vi "ANA IN Lesen.vi"() -> (0 "Rohwerte":sgl[](array[numeric]), 1 "Istwerte":sgl[](array[numeric]), 3 "Fühlerbruch":bool[](array[boolean]))   [LabVIEW 2020, in "Verwaltung - cRIO.lvlib"]
uses:
  Verwaltung - cRIO.lvlib
  Konfig-Dateien/FGV Betriebsdaten Aktionen.ctl
  Allgemein/FGV FT-IR Kuehlung Aktionen.ctl
  Allgemein/Allgemein.lvlib
  Konfig-Dateien/Konfig-Dateien.lvlib
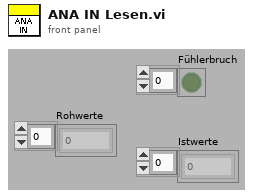
[diagram p1: front panel]
types:
  T1 = typedef "Allgemein.lvlib/FGV FT-IR Kuehlung Aktionen.ctl" = enum16{"lesen", "Kühlung?"}
  T2 = typedef "Konfig-Dateien.lvlib/FGV Betriebsdaten Aktionen.ctl" = enum16{"lesen", "Anlagengrenzw.", "PID Param.", "Sonstige", "Sensor Para."}
  T3 = typedef "Erweiterte Konfig.lvlib/Parameter Sensoren.ctl" = cluster{"Kal.Durchfl.FTIR":sgl, "Kal.Durchfl.PMA":sgl, "Offset Durchfl.FTIR":sgl, "Offset Druck Ausgang":sgl, "Offset Druck Umgebung":sgl, "Offset Durchfl.PMA":sgl, "Offset Druck CG PMA":sgl, "Offset Druck CG":sgl, "Offset Druck FTIR IAG":sgl, "Druck Kalter Block":sgl}
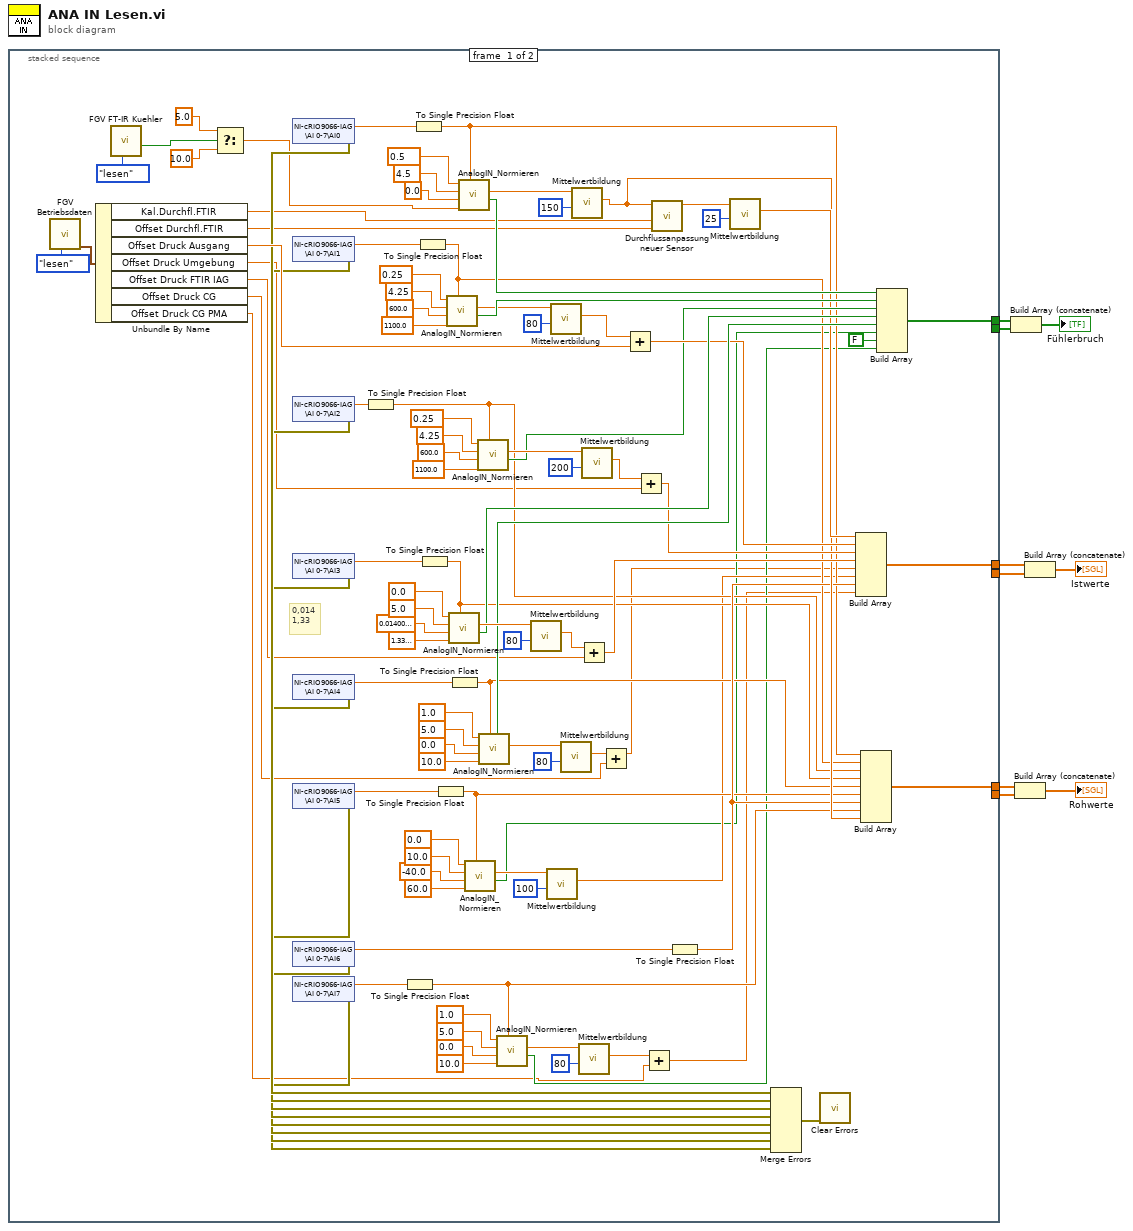
[diagram p0: block diagram]
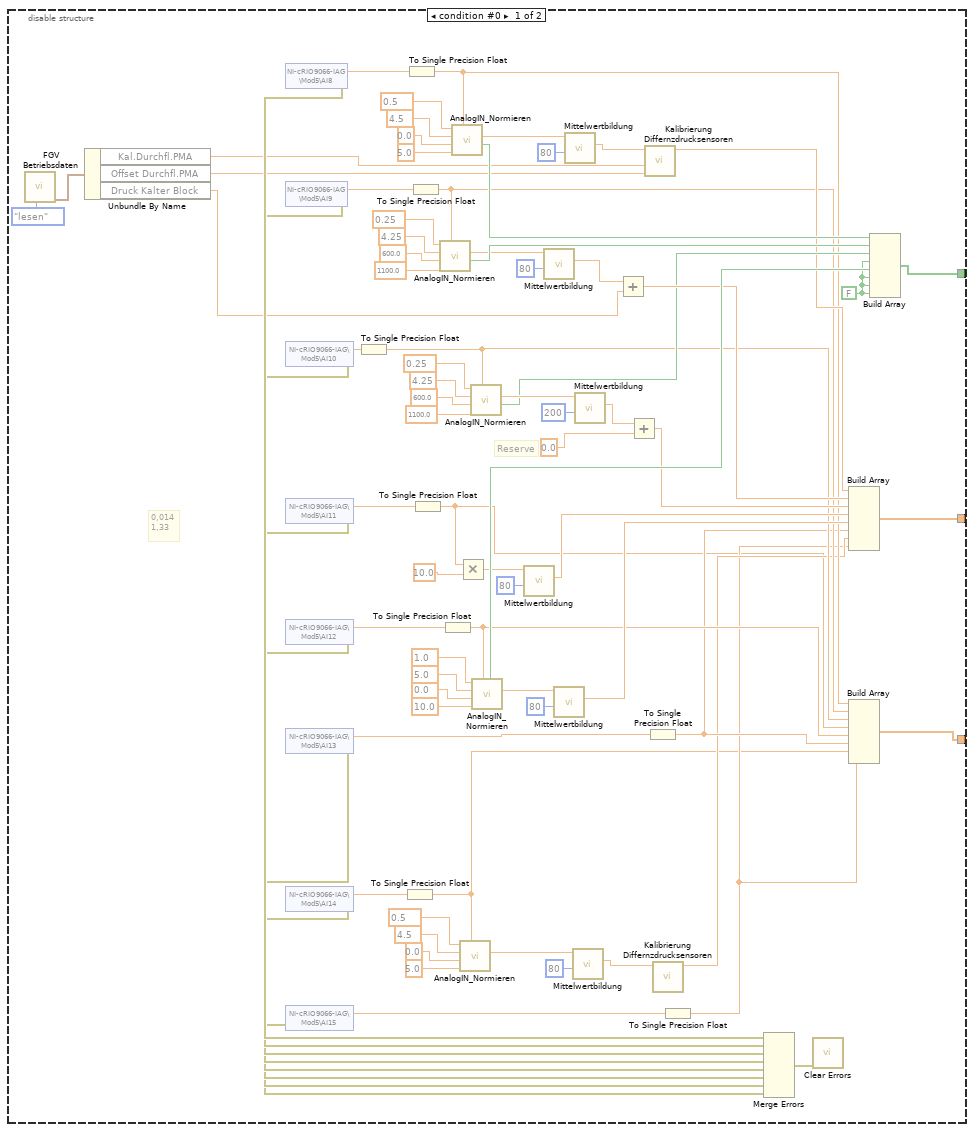
[diagram p3: hidden frame]
diagram:
  n1 = stacked-sequence {
    tunnel: [w50 _] -> w9
    tunnel: [_ w118] -> w8
    tunnel: [w49 _] -> w7
    tunnel: [_ w117] -> w6
    tunnel: [w42 _] -> w2
    tunnel: [_ w116] -> w3
    frame #0 {
      # "0,014\n1,33"
      n2 = call "FGV Betriebsdaten.vi"("Aktionen"=FGV_Betriebsdaten_Aktionen."lesen") -> ("Parameter Sensoren"=w21:T3)  [unwired: 7 in, 3 out]
      n3 = Unbundle By Name(w21) -> ("Kal.Durchfl.FTIR"=w55:sgl, "Offset Durchfl.FTIR"=w54:sgl, "Offset Druck Ausgang"=w77:sgl, "Offset Druck Umgebung"=w20:sgl, "Offset Druck FTIR IAG"=w19:sgl, "Offset Druck CG"=w17:sgl, "Offset Druck CG PMA"=w15:sgl)
      n4 = call "FGV FT-IR Kuehler.vi"("Aktionen"=FGV_FT-IR_Kuehlung_Aktionen."lesen") -> ("Durchflusssensor 0-5V"=w11:bool)  [unwired: 6 in, 4 out]
      n5 = Select(t=sgl 5.0 ("Obergrenze"), s=w11, f=sgl 10.0 ("Obergrenze")) -> (s? t:f=w10:sgl)
      n6 = shared-variable "NI-cRIO9066-IAG\\AI 0-7\\AI0"() -> (w101:dbl, error out=w73:errorcluster)  [unwired: 1 in]
      n7 = shared-variable "NI-cRIO9066-IAG\\AI 0-7\\AI1"() -> (w100:dbl, error out=w72:errorcluster)  [unwired: 1 in]
      n8 = shared-variable "NI-cRIO9066-IAG\\AI 0-7\\AI2"() -> (w99:dbl, error out=w71:errorcluster)  [unwired: 1 in]
      n9 = shared-variable "NI-cRIO9066-IAG\\AI 0-7\\AI3"() -> (w97:dbl, error out=w70:errorcluster)  [unwired: 1 in]
      n10 = shared-variable "NI-cRIO9066-IAG\\AI 0-7\\AI4"() -> (w85:dbl, error out=w69:errorcluster)  [unwired: 1 in]
      n11 = shared-variable "NI-cRIO9066-IAG\\AI 0-7\\AI5"() -> (w35:dbl, error out=w68:errorcluster)  [unwired: 1 in]
      n12 = shared-variable "NI-cRIO9066-IAG\\AI 0-7\\AI6"() -> (w83:dbl, error out=w67:errorcluster)  [unwired: 1 in]
      n13 = shared-variable "NI-cRIO9066-IAG\\AI 0-7\\AI7"() -> (w82:dbl, error out=w66:errorcluster)  [unwired: 1 in]
      n14 = To Single Precision Float(number=w99) -> (single precision float=w45:sgl)
      n15 = To Single Precision Float(number=w82) -> (single precision float=w25:sgl)
      n16 = To Single Precision Float(number=w101) -> (single precision float=w43:sgl)
      n17 = To Single Precision Float(number=w100) -> (single precision float=w44:sgl)
      n18 = To Single Precision Float(number=w97) -> (single precision float=w46:sgl)
      n19 = To Single Precision Float(number=w35) -> (single precision float=w34:sgl)
      n20 = call "AnalogIN_Normieren.vi"("Analogwert"=w44, "Obergrenze"=sgl 1100.0, "Untergrenze"=sgl 600.0, "Max Analogwert"=sgl 4.25, "Min Analogwert"=sgl 0.25) -> ("Unterlauf oder Drahtbruch"=w115:bool, "Normierter Wert"=w102:sgl)  [unwired: 5 out]
      n21 = call "AnalogIN_Normieren.vi"("Analogwert"=w46, "Obergrenze"=sgl 1.33 ("Max Analogwert"), "Untergrenze"=sgl 0.014 ("Min Analogwert"), "Max Analogwert"=sgl 5.0, "Min Analogwert"=sgl 0.0) -> ("Unterlauf oder Drahtbruch"=w81:bool, "Normierter Wert"=w92:sgl)  [unwired: 5 out]
      n22 = To Single Precision Float(number=w85) -> (single precision float=w33:sgl)
      n23 = call "AnalogIN_Normieren.vi"("Analogwert"=w43, "Obergrenze"=w10, "Untergrenze"=sgl 0.0, "Max Analogwert"=sgl 4.5, "Min Analogwert"=sgl 0.5) -> ("Unterlauf oder Drahtbruch"=w114:bool, "Normierter Wert"=w103:sgl)  [unwired: 5 out]
      n24 = call "AnalogIN_Normieren.vi"("Analogwert"=w34, "Obergrenze"=sgl 60.0 ("Max Analogwert"), "Untergrenze"=sgl -40.0 ("Min Analogwert"), "Max Analogwert"=sgl 10.0, "Min Analogwert"=sgl 0.0) -> ("Unterlauf oder Drahtbruch"=w23:bool, "Normierter Wert"=w36:sgl)  [unwired: 5 out]
      n25 = call "AnalogIN_Normieren.vi"("Analogwert"=w45, "Obergrenze"=sgl 1100.0, "Untergrenze"=sgl 600.0, "Max Analogwert"=sgl 4.25, "Min Analogwert"=sgl 0.25) -> ("Unterlauf oder Drahtbruch"=w58:bool, "Normierter Wert"=w64:sgl)  [unwired: 5 out]
      n26 = call "AnalogIN_Normieren.vi"("Analogwert"=w33, "Obergrenze"=sgl 10.0 ("Max Analogwert"), "Untergrenze"=sgl 0.0 ("Min Analogwert"), "Max Analogwert"=sgl 5.0, "Min Analogwert"=sgl 1.0) -> ("Unterlauf oder Drahtbruch"=w80:bool, "Normierter Wert"=w91:sgl)  [unwired: 5 out]
      n27 = call "AnalogIN_Normieren.vi"("Analogwert"=w25, "Obergrenze"=sgl 10.0 ("Max Analogwert"), "Untergrenze"=sgl 0.0 ("Min Analogwert"), "Max Analogwert"=sgl 5.0, "Min Analogwert"=sgl 1.0) -> ("Unterlauf oder Drahtbruch"=w22:bool, "Normierter Wert"=w27:sgl)  [unwired: 5 out]
      n28 = call "Mittelwertbildung.vi"("Anzahl Werte"=u8 80, "Neuer Wert"=w92) -> ("gemittelter Wert"=w76:sgl)  [unwired: 7 in, 2 out]
      n29 = call "Mittelwertbildung.vi"("Anzahl Werte"=u8 100, "Neuer Wert"=w36) -> ("gemittelter Wert"=w24:sgl)  [unwired: 7 in, 2 out]
      n30 = call "Mittelwertbildung.vi"("Anzahl Werte"=u8 80, "Neuer Wert"=w102) -> ("gemittelter Wert"=w79:sgl)  [unwired: 7 in, 2 out]
      n31 = call "Mittelwertbildung.vi"("Anzahl Werte"=u8 80, "Neuer Wert"=w91) -> ("gemittelter Wert"=w84:sgl)  [unwired: 7 in, 2 out]
      n32 = call "Mittelwertbildung.vi"("Anzahl Werte"=u8 150, "Neuer Wert"=w103) -> ("gemittelter Wert"=w48:sgl)  [unwired: 7 in, 2 out]
      n33 = Add(x=w76, y=w19) -> (x+y=w75:sgl)
      n34 = call "Mittelwertbildung.vi"("Anzahl Werte"=u8 80, "Neuer Wert"=w27) -> ("gemittelter Wert"=w26:sgl)  [unwired: 7 in, 2 out]
      n35 = call "Mittelwertbildung.vi"("Anzahl Werte"=u8 200, "Neuer Wert"=w64) -> ("gemittelter Wert"=w57:sgl)  [unwired: 7 in, 2 out]
      n36 = Add(x=w84, y=w17) -> (x+y=w18:sgl)
      n37 = Add(x=w79, y=w77) -> (x+y=w78:sgl)
      n38 = Add(x=w57, y=w20) -> (x+y=w56:sgl)
      n39 = Add(x=w26, y=w15) -> (x+y=w16:sgl)
      n40 = call "Durchflussanpassung neuer Sensor.vi"("Offset"=w54, "Endpunkt"=w55, "Eingang"=w48) -> ("Ausgang"=w52:dbl)  [unwired: 8 in]
      n41 = To Single Precision Float(number=w83) -> (single precision float=w47:sgl)
      n42 = call "Mittelwertbildung.vi"("Anzahl Werte"=u8 25, "Neuer Wert"=w52) -> ("gemittelter Wert"=w51:sgl)  [unwired: 7 in, 2 out]
      n43 = Merge Errors(w73, w72, w71, w70, w69, w68, w67, w66) -> (w65:errorcluster)
      n44 = call <vilib>:"Clear Errors.vi"("error in (no error)"=w65) -> ()  [unwired: 5 in, 2 out]
      n45 = Build Array(w51, w78, w56, w75, w18, w24, w47, w16) -> (w49:sgl[])
      n46 = Build Array(w43, w44, w45, w46, w33, w34, w47, w25, w48) -> (w42:sgl[])
      n47 = Build Array(w114, w115, w58, w81, w80, w23, FALSE ("Element"), w22) -> (w50:bool[])
    }
    frame #1 {
      n48 = disable-structure shown="PMA==FALSE, Standard" {
        disable-tunnel: [w144 _] -> w118
        disable-tunnel: [w143 _] -> w117
        disable-tunnel: [w135 _] -> w116
        frame condition #0 {
          w134 = FALSE ("Element")
          # "Reserve"
          # "0,014\n1,33"
          n49 = call "FGV Betriebsdaten.vi"("Aktionen"=FGV_Betriebsdaten_Aktionen."lesen") -> ("Parameter Sensoren"=w130:T3)  [unwired: 7 in, 3 out]
          n50 = Unbundle By Name(w130) -> ("Kal.Durchfl.PMA"=w148:sgl, "Offset Durchfl.PMA"=w147:sgl, "Druck Kalter Block"=w119:sgl)
          n51 = shared-variable "NI-cRIO9066-IAG\\Mod5\\AI8"() -> (w186:dbl, error out=w166:errorcluster)  [unwired: 1 in]
          n52 = shared-variable "NI-cRIO9066-IAG\\Mod5\\AI9"() -> (w185:dbl, error out=w165:errorcluster)  [unwired: 1 in]
          n53 = shared-variable "NI-cRIO9066-IAG\\Mod5\\AI10"() -> (w184:dbl, error out=w164:errorcluster)  [unwired: 1 in]
          n54 = shared-variable "NI-cRIO9066-IAG\\Mod5\\AI11"() -> (w183:dbl, error out=w163:errorcluster)  [unwired: 1 in]
          n55 = shared-variable "NI-cRIO9066-IAG\\Mod5\\AI12"() -> (w175:dbl, error out=w162:errorcluster)  [unwired: 1 in]
          n56 = shared-variable "NI-cRIO9066-IAG\\Mod5\\AI13"() -> (w173:dbl, error out=w161:errorcluster)  [unwired: 1 in]
          n57 = shared-variable "NI-cRIO9066-IAG\\Mod5\\AI14"() -> (w122:dbl, error out=w160:errorcluster)  [unwired: 1 in]
          n58 = shared-variable "NI-cRIO9066-IAG\\Mod5\\AI15"() -> (w172:dbl, error out=w159:errorcluster)  [unwired: 1 in]
          n59 = To Single Precision Float(number=w184) -> (single precision float=w140:sgl)
          n60 = To Single Precision Float(number=w122) -> (single precision float=w121:sgl)
          n61 = To Single Precision Float(number=w186) -> (single precision float=w142:sgl)
          n62 = To Single Precision Float(number=w185) -> (single precision float=w141:sgl)
          n63 = To Single Precision Float(number=w183) -> (single precision float=w132:sgl)
          n64 = call "AnalogIN_Normieren.vi"("Analogwert"=w141, "Obergrenze"=sgl 1100.0, "Untergrenze"=sgl 600.0, "Max Analogwert"=sgl 4.25, "Min Analogwert"=sgl 0.25) -> ("Unterlauf oder Drahtbruch"=w200:bool, "Normierter Wert"=w187:sgl)  [unwired: 5 out]
          n65 = To Single Precision Float(number=w175) -> (single precision float=w139:sgl)
          n66 = call "AnalogIN_Normieren.vi"("Analogwert"=w142, "Obergrenze"=sgl 5.0, "Untergrenze"=sgl 0.0, "Max Analogwert"=sgl 4.5, "Min Analogwert"=sgl 0.5) -> ("Unterlauf oder Drahtbruch"=w199:bool, "Normierter Wert"=w188:sgl)  [unwired: 5 out]
          n67 = Multiply(x=w132, y=sgl 10.0 ("x")) -> (x*y=w131:sgl)
          n68 = call "AnalogIN_Normieren.vi"("Analogwert"=w121, "Obergrenze"=sgl 5.0, "Untergrenze"=sgl 0.0, "Max Analogwert"=sgl 4.5, "Min Analogwert"=sgl 0.5) -> ("Normierter Wert"=w128:sgl)  [unwired: 6 out]
          n69 = call "AnalogIN_Normieren.vi"("Analogwert"=w140, "Obergrenze"=sgl 1100.0, "Untergrenze"=sgl 600.0, "Max Analogwert"=sgl 4.25, "Min Analogwert"=sgl 0.25) -> ("Unterlauf oder Drahtbruch"=w151:bool, "Normierter Wert"=w157:sgl)  [unwired: 5 out]
          n70 = call "AnalogIN_Normieren.vi"("Analogwert"=w139, "Obergrenze"=sgl 10.0 ("Max Analogwert"), "Untergrenze"=sgl 0.0 ("Min Analogwert"), "Max Analogwert"=sgl 5.0, "Min Analogwert"=sgl 1.0) -> ("Unterlauf oder Drahtbruch"=w171:bool, "Normierter Wert"=w181:sgl)  [unwired: 5 out]
          n71 = call "Mittelwertbildung.vi"("Anzahl Werte"=u8 80, "Neuer Wert"=w131) -> ("gemittelter Wert"=w168:sgl)  [unwired: 7 in, 2 out]
          n72 = call "Mittelwertbildung.vi"("Anzahl Werte"=u8 80, "Neuer Wert"=w187) -> ("gemittelter Wert"=w170:sgl)  [unwired: 7 in, 2 out]
          n73 = call "Mittelwertbildung.vi"("Anzahl Werte"=u8 80, "Neuer Wert"=w181) -> ("gemittelter Wert"=w174:sgl)  [unwired: 7 in, 2 out]
          n74 = call "Mittelwertbildung.vi"("Anzahl Werte"=u8 80, "Neuer Wert"=w188) -> ("gemittelter Wert"=w145:sgl)  [unwired: 7 in, 2 out]
          n75 = call "Mittelwertbildung.vi"("Anzahl Werte"=u8 80, "Neuer Wert"=w128) -> ("gemittelter Wert"=w129:sgl)  [unwired: 7 in, 2 out]
          n76 = call "Mittelwertbildung.vi"("Anzahl Werte"=u8 200, "Neuer Wert"=w157) -> ("gemittelter Wert"=w150:sgl)  [unwired: 7 in, 2 out]
          n77 = Add(x=w170, y=w119) -> (x+y=w169:sgl)
          n78 = Add(x=w150, y=0.0) -> (x+y=w149:dbl)
          n79 = call "Kalibrierung Differnzdrucksensoren.vi"("Nullpunktverschiebung"=w147, "Kalibrierter Wert"=w148, "Normierter Wert"=w145) -> ("Kalibrierter Wert"=w146:sgl)  [unwired: 8 in]
          n80 = To Single Precision Float(number=w173) -> (single precision float=w138:sgl)
          n81 = call "Kalibrierung Differnzdrucksensoren.vi"("Normierter Wert"=w129) -> ("Kalibrierter Wert"=w137:sgl)  [unwired: 10 in]
          n82 = To Single Precision Float(number=w172) -> (single precision float=w136:sgl)
          n83 = Merge Errors(w166, w165, w164, w163, w162, w161, w160, w159) -> (w158:errorcluster)
          n84 = call <vilib>:"Clear Errors.vi"("error in (no error)"=w158) -> ()  [unwired: 5 in, 2 out]
          n85 = Build Array(w146, w169, w149, w168, w174, w138, w137, w136) -> (w143:dbl[])
          n86 = Build Array(w142, w141, w140, w132, w139, w138, w121, w136) -> (w135:sgl[])
          n87 = Build Array(w199, w200, w151, w134, w171, w134, w134, w134) -> (w144:bool[])
        }
        frame condition #1 (active) {
        }
      }
    }
  }
  n88 = Build Array (concatenate)(w9, w8) -> (→"Fühlerbruch":bool[])
  n89 = Build Array (concatenate)(w2, w3) -> (→"Rohwerte":sgl[])
  n90 = Build Array (concatenate)(w7, w6) -> (→"Istwerte":dbl[])
